vi "pAmp_HISTO_GET.vi"(0 "TCP Network Connection in":refnum<k5>, 5 "error in (no error)":errorcluster) -> (14 "TCP Network Connection out":refnum<k5>, 15 "BINS_N":u32, 16 "Oscilloscope":u32[](graph), 17 "DONE":u32, 18 "CURR_COUNT":u32, 19 "error out":errorcluster)   [LabVIEW 2019, in "Histogram.lvlib"]
uses:
  Histogram.lvlib
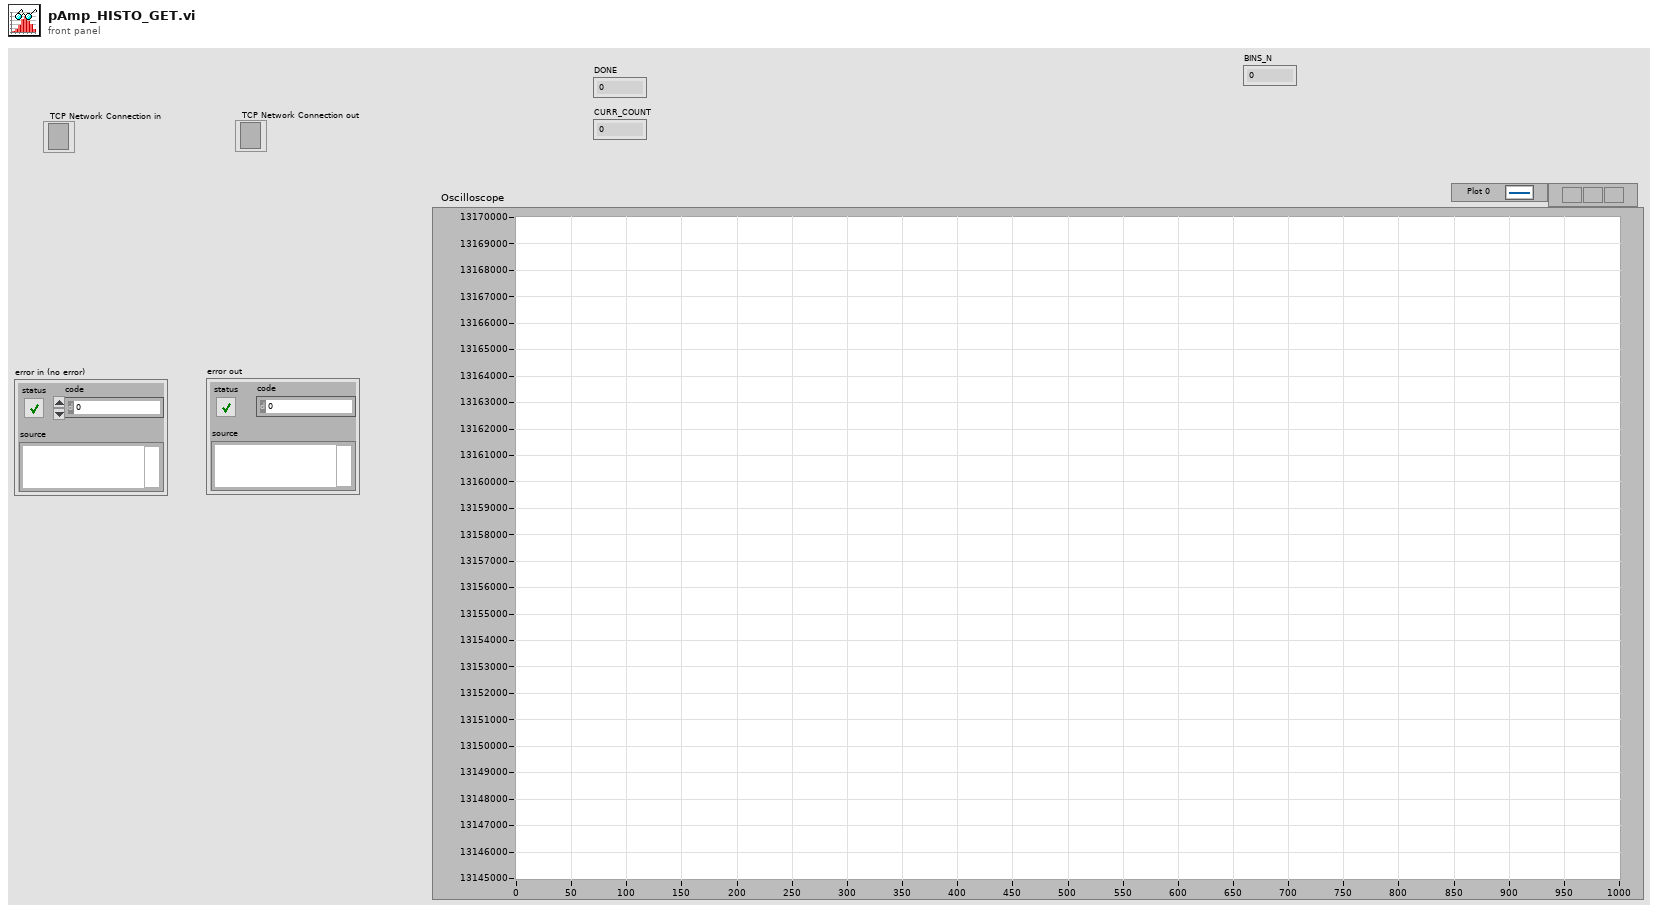
[diagram p1: front panel]
types:
  T1 = enum16{"big-endian, network order", "native, host order", "little-endian"}
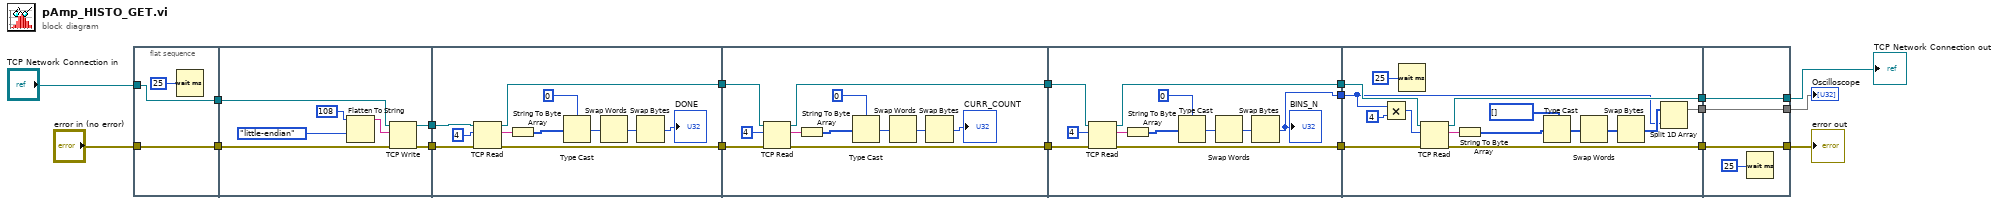
[diagram p0: block diagram]
diagram:
  n1 = flat-sequence {
    tunnel: [w21] -> w15
    tunnel: [w22] -> w14
    tunnel: "error in (no error)" -> [w22]
    tunnel: "TCP Network Connection in" -> [w21]
    tunnel: w15 -> [w29]
    tunnel: w14 -> [w28]
    tunnel: [w27] -> w9
    tunnel: [w26] -> w8
    tunnel: w9 -> [w37]
    tunnel: w8 -> [w40]
    tunnel: [w39] -> w7
    tunnel: [w38] -> w6
    tunnel: w7 -> [w44]
    tunnel: w6 -> [w45]
    tunnel: [w43] -> w5
    tunnel: [w42] -> w4
    tunnel: w5 -> [w56]
    tunnel: w4 -> [w55]
    tunnel: [w54] -> w3
    tunnel: [w53] -> w2
    tunnel: [w52] -> w1
    tunnel: [w75] -> w12
    tunnel: [w74] -> w11
    tunnel: [w65] -> w10
    tunnel: w3 -> [w77]
    tunnel: w2 -> [w76]
    tunnel: w1 -> [w64]
    tunnel: [w79] -> w13
    tunnel: [w80] -> w17
    tunnel: [w81] -> w16
    tunnel: w12 -> [w81]
    tunnel: w11 -> [w80]
    tunnel: w10 -> [w79]
    frame #0 {
      n2 = Wait (ms)(milliseconds to wait=u32 25) -> ()  [unwired: 1 out]
    }
    frame #1 {
      n3 = Flatten To String(anything=u32 108 ("element"), byte order (0:big-endian, network order)=T1."little-endian") -> (data string=w23:string)  [unwired: 2 in, 2 out]
      n4 = TCP Write(connection ID=w29, data in=w23, error in (no error)=w28) -> (connection ID out=w27:refnum<k5>, error out=w26:errorcluster)  [unwired: 1 in, 1 out]
    }
    frame #2 {
      n5 = TCP Read(connection ID=w37, bytes to read=4, error in (no error)=w40) -> (connection ID out=w38:refnum<k5>, data out=w36:string, error out=w39:errorcluster)  [unwired: 2 in]
      n6 = String To Byte Array(string=w36) -> (unsigned byte array=w34:u8[])
      n7 = Type Cast(type=u32 0 ("y"), x=w34) -> (*(type *) &x=w33:u32)
      n8 = Swap Words(1:w33) -> (0:w32:u32)
      n9 = Swap Bytes(anything=w32) -> (byte swapped=→"DONE":u32)
    }
    frame #3 {
      n10 = TCP Read(connection ID=w45, bytes to read=4, error in (no error)=w44) -> (connection ID out=w43:refnum<k5>, data out=w51:string, error out=w42:errorcluster)  [unwired: 2 in]
      n11 = String To Byte Array(string=w51) -> (unsigned byte array=w49:u8[])
      n12 = Type Cast(type=u32 0 ("y"), x=w49) -> (*(type *) &x=w48:u32)
      n13 = Swap Words(1:w48) -> (0:w47:u32)
      n14 = Swap Bytes(anything=w47) -> (byte swapped=→"CURR_COUNT":u32)
    }
    frame #4 {
      n15 = TCP Read(connection ID=w56, bytes to read=4, error in (no error)=w55) -> (connection ID out=w54:refnum<k5>, data out=w62:string, error out=w53:errorcluster)  [unwired: 2 in]
      n16 = String To Byte Array(string=w62) -> (unsigned byte array=w60:u8[])
      n17 = Type Cast(type=u32 0 ("y"), x=w60) -> (*(type *) &x=w59:u32)
      n18 = Swap Words(1:w59) -> (0:w58:u32)
      n19 = Swap Bytes(anything=w58) -> (byte swapped=w52:u32)
      "BINS_N" <- w52
    }
    frame #5 {
      n20 = Multiply(x=w64, y=u32 4) -> (x*y=w72:u32)
      n21 = Wait (ms)(milliseconds to wait=u32 25) -> ()  [unwired: 1 out]
      n22 = TCP Read(connection ID=w77, bytes to read=w72, error in (no error)=w76) -> (connection ID out=w75:refnum<k5>, data out=w63:string, error out=w74:errorcluster)  [unwired: 2 in]
      n23 = String To Byte Array(string=w63) -> (unsigned byte array=w70:u8[])
      n24 = Type Cast(type=u32[] [], x=w70) -> (*(type *) &x=w68:u32[])
      n25 = Swap Words(1:w68) -> (0:w67:u32[])
      n26 = Swap Bytes(anything=w67) -> (byte swapped=w66:u32[])
      n27 = Split 1D Array(array=w66, index=w64) -> (first subarray=w65:u32[])  [unwired: 1 out]
    }
    frame #6 {
      n28 = Wait (ms)(milliseconds to wait=u32 25) -> ()  [unwired: 1 out]
    }
  }
  "error out" <- w17
  "TCP Network Connection out" <- w16
  "Oscilloscope" <- w13
